vi "Unflatten.vi"(8 "error in":errorcluster, 10 "Buffer":u8[](array[numeric]) format="%.0x") -> (0 "error out":errorcluster, 2 "Data":T1)   [LabVIEW 2020, in "Discovery.lvlib"]
uses:
  Discovery.lvlib
  Data.ctl
  lv-protoc/LV-Proto/Wire Decode Varint I32.vi
  lv-protoc/LV-Proto/Extract Varint Bytes.vi
  lv-protoc/LV-Proto/LV-Proto.lvlib
  ServiceType/Enumeration.ctl
  ServiceType/ServiceType.lvlib
  Service/Data.ctl
  Service/Service.lvlib
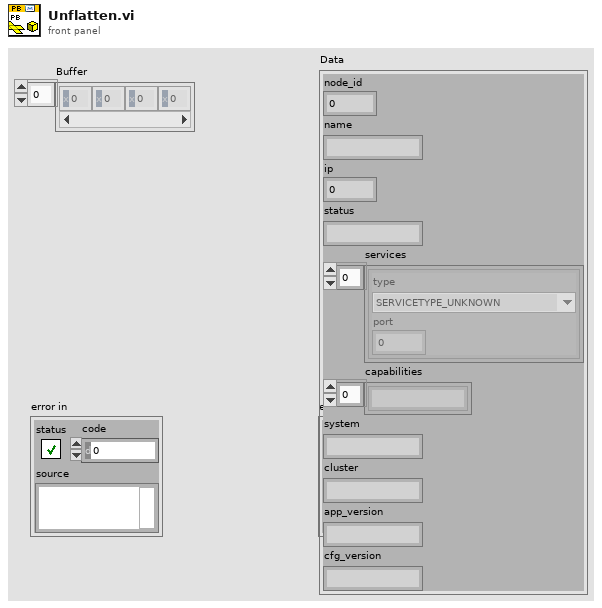
[diagram p1: front panel]
types:
  T1 = typedef "Discovery.lvlib/Data.ctl" = cluster{"node_id":u32, "name":string, "ip":u32, "status":string, "services":T2[], "capabilities":string[], "system":string, "cluster":string, "app_version":string, "cfg_version":string}
  T2 = typedef "Service.lvlib/Data.ctl" = cluster{"type":T3, "port":i32}
  T3 = typedef "ServiceType.lvlib/Enumeration.ctl" = enum16{"SERVICETYPE_UNKNOWN", "SERVICETYPE_TCPSERVER", "SERVICETYPE_HTTPSERVER"}
  T4 = typedef "LV-Proto.lvlib/Wire Type.ctl" = enum8{"VARINT", "I64", "LEN", "SGROUP (Deprecated)", "EGROUP (Deprecated)", "I32"}
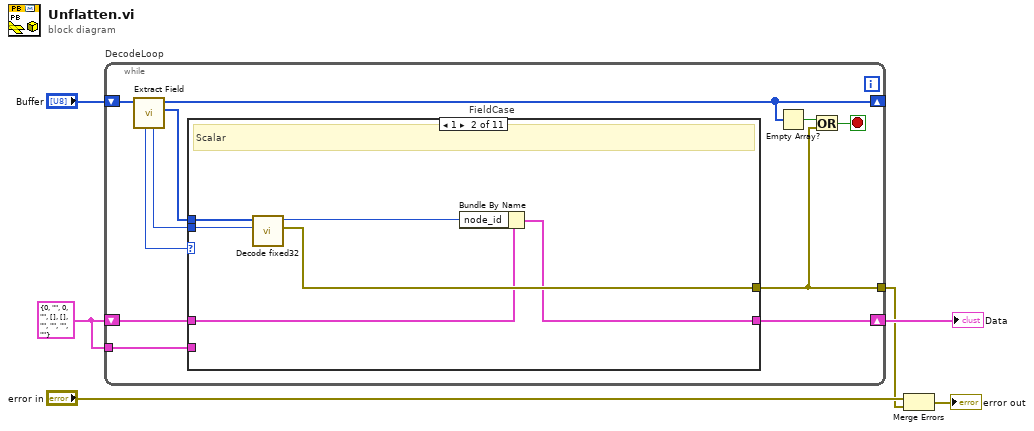
[diagram p0: block diagram]
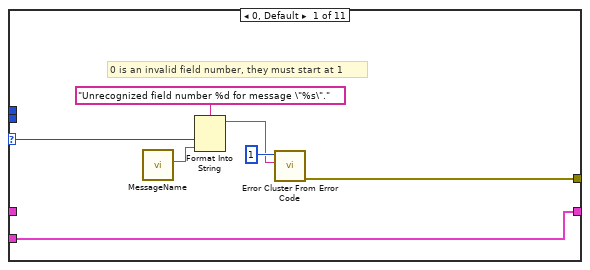
[diagram p2: hidden frame]
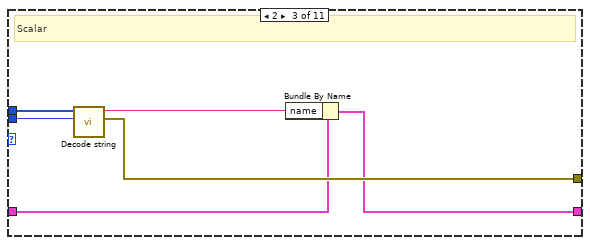
[diagram p3: hidden frame]
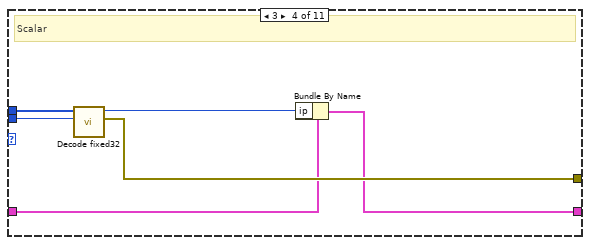
[diagram p4: hidden frame]
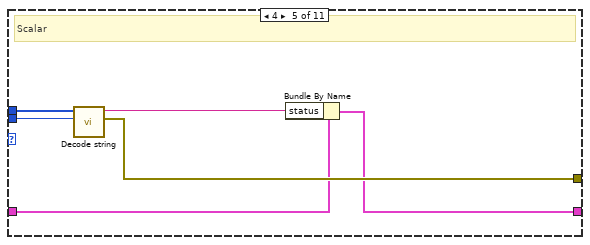
[diagram p5: hidden frame]
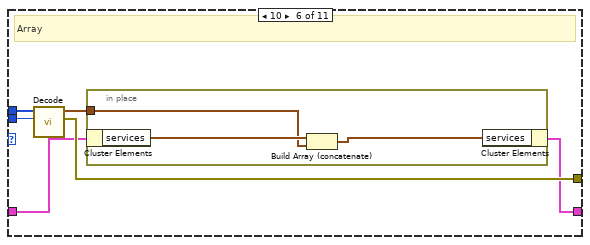
[diagram p6: hidden frame]
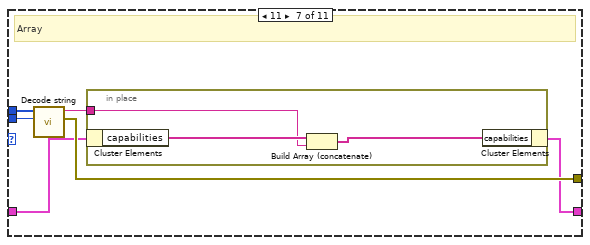
[diagram p7: hidden frame]
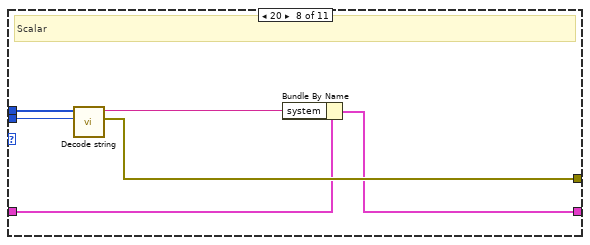
[diagram p8: hidden frame]
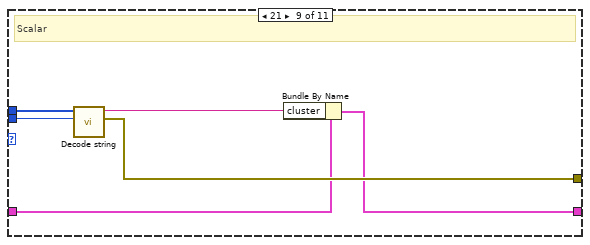
[diagram p9: hidden frame]
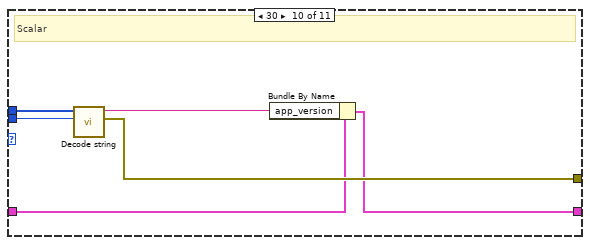
[diagram p10: hidden frame]
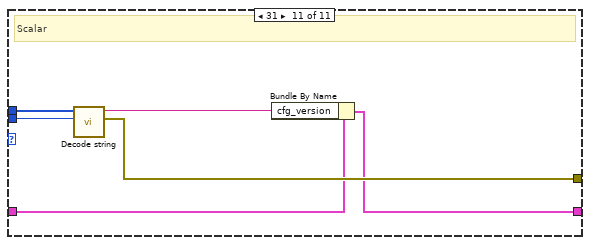
[diagram p11: hidden frame]
diagram:
  w4 = T1 {"node_id"=0, "name"="", "ip"=0, "status"="", "services"=[], "capabilities"=[], "system"="", "cluster"="", "app_version"="", "cfg_version"=""} ("Data")
  n1 = while "DecodeLoop" {
    shift-right: [w16] -> _
    shift-left: "Buffer" -> [w17]
    shift-right: [w9] -> w5
    shift-left: w4 -> [w15]
    tunnel: [w8] -> w2
    tunnel: w4 -> [w7]
    stop <- w11 stop-if-true
    n2 = call "Extract Field.vi"("Buffer in"=w17) -> ("Field Data"=w10:u8[], "Buffer"=w16:u8[], "Wire Type"=w13:T4, "Field Number"=w14:i32)  [unwired: 7 in]
    n3 = case "FieldCase" shown="1" w14 {
      selector: w14 -> [w23 _ _ _ _ _ _ _ _ _ _]
      tunnel: w15 -> [_ w26 w32 w38 w44 w51 w60 w68 w74 w80 w86]
      tunnel: w13 -> [_ w28 w34 w40 w46 w52 w61 w70 w76 w82 w88]
      tunnel: w10 -> [_ w29 w35 w41 w47 w53 w62 w71 w77 w83 w89]
      tunnel: [w19 w25 w31 w37 w43 w50 w59 w67 w73 w79 w85] -> w9
      tunnel: [w20 w30 w36 w42 w48 w54 w63 w72 w78 w84 w90] -> w8
      tunnel: w7 -> [w19 _ _ _ _ _ _ _ _ _ _]
      frame 0, Default {
        # "0 is an invalid field number, they must start at 1"
        n4 = call "MessageName.vi"() -> ("MessageName"=w18:string)  [unwired: 11 in]
        n5 = Format Into String(format string="Unrecognized field number %d for message \"%s\".", w23, w18) -> (resulting string=w21:string)  [unwired: 2 in, 1 out]
        n6 = call <vilib>:"Error Cluster From Error Code.vi"("error message (\"\")"=w21, "error code (0)"=1) -> ("error out"=w20:errorcluster)  [unwired: 7 in]
      }
      frame 1 {
        # "Scalar"
        n7 = call "Decode fixed32.vi"("Wire Type"=w28, "Data"=w29) -> ("error out"=w30:errorcluster, "fixed32"=w27:u32)  [unwired: 8 in]
        n8 = Bundle By Name(cluster=w26, "node_id"=w27) -> (w25:T1)
      }
      frame 2 {
        # "Scalar"
        n9 = call "Decode string.vi"("Wire Type"=w34, "Data"=w35) -> ("error out"=w36:errorcluster, "string"=w33:string)  [unwired: 8 in]
        n10 = Bundle By Name(cluster=w32, "name"=w33) -> (w31:T1)
      }
      frame 3 {
        # "Scalar"
        n11 = call "Decode fixed32.vi"("Wire Type"=w40, "Data"=w41) -> ("error out"=w42:errorcluster, "fixed32"=w39:u32)  [unwired: 8 in]
        n12 = Bundle By Name(cluster=w38, "ip"=w39) -> (w37:T1)
      }
      frame 4 {
        # "Scalar"
        n13 = call "Decode string.vi"("Wire Type"=w46, "Data"=w47) -> ("error out"=w48:errorcluster, "string"=w45:string)  [unwired: 8 in]
        n14 = Bundle By Name(cluster=w44, "status"=w45) -> (w43:T1)
      }
      frame 10 {
        # "Array"
        n15 = call "Decode.vi"("Wire Type"=w52, "Buffer"=w53) -> ("error out"=w54:errorcluster, "Data"=w49:T2)  [unwired: 8 in]
        n16 = in-place {
          in-place-border: w49 -> [w55]
          n17 = in-place-cluster #1(w51) -> ("services"=w57:T2[])
          n18 = Build Array (concatenate)(w57, w55) -> (w56:T2[])
          n19 = in-place-cluster #1("services"=w56) -> (w50:T1)
        }
      }
      frame 11 {
        # "Array"
        n20 = call "Decode string.vi"("Wire Type"=w61, "Data"=w62) -> ("error out"=w63:errorcluster, "string"=w58:string)  [unwired: 8 in]
        n21 = in-place {
          in-place-border: w58 -> [w64]
          n22 = in-place-cluster #2(w60) -> ("capabilities"=w66:string[])
          n23 = Build Array (concatenate)(w66, w64) -> (w65:string[])
          n24 = in-place-cluster #2("capabilities"=w65) -> (w59:T1)
        }
      }
      frame 20 {
        # "Scalar"
        n25 = call "Decode string.vi"("Wire Type"=w70, "Data"=w71) -> ("error out"=w72:errorcluster, "string"=w69:string)  [unwired: 8 in]
        n26 = Bundle By Name(cluster=w68, "system"=w69) -> (w67:T1)
      }
      frame 21 {
        # "Scalar"
        n27 = call "Decode string.vi"("Wire Type"=w76, "Data"=w77) -> ("error out"=w78:errorcluster, "string"=w75:string)  [unwired: 8 in]
        n28 = Bundle By Name(cluster=w74, "cluster"=w75) -> (w73:T1)
      }
      frame 30 {
        # "Scalar"
        n29 = call "Decode string.vi"("Wire Type"=w82, "Data"=w83) -> ("error out"=w84:errorcluster, "string"=w81:string)  [unwired: 8 in]
        n30 = Bundle By Name(cluster=w80, "app_version"=w81) -> (w79:T1)
      }
      frame 31 {
        # "Scalar"
        n31 = call "Decode string.vi"("Wire Type"=w88, "Data"=w89) -> ("error out"=w90:errorcluster, "string"=w87:string)  [unwired: 8 in]
        n32 = Bundle By Name(cluster=w86, "cfg_version"=w87) -> (w85:T1)
      }
    }
    n33 = Empty Array?(array=w16) -> (empty?=w12:bool)
    n34 = Or(x=w12, y=w8) -> (x .or. y?=w11:bool)
  }
  "Data" <- w5
  n35 = Merge Errors("error in", w2) -> (→"error out":errorcluster)
